vi "Configure Session.vi"(8 "error in":errorcluster, 11 "Plugin in":refnum<class "Statistic.lvclass">) -> (0 "error out":errorcluster, 3 "Plugin out":refnum<class "Statistic.lvclass">)   [LabVIEW 2025, in "Statistic.lvlib" / "Statistic.lvclass"]
uses:
  Statistic.lvclass
  C:/Program Files/National Instruments/LabVIEW 2025/vi.lib/FlexLogger/SDK/PluginSDK.lvlibp/PEFClasses/SDK/Plugin/Plugin.lvclass
  Statistic.lvclass/Statistic.ctl
  <vilib>/FlexLogger/SDK/PluginSDK.lvlibp/PEFClasses/SDK/Producer Channel/Producer Channel.lvclass
  C:/Program Files/National Instruments/LabVIEW 2025/vi.lib/FlexLogger/SDK/PluginSDK.lvlibp/PEFClasses/SDK/Channel/Channel.lvclass
  <vilib>/FlexLogger/SDK/PluginSDK.lvlibp/PEFClasses/SDK/Plugin/ParameterAccess/Read Boolean.vi
  <vilib>/FlexLogger/SDK/PluginSDK.lvlibp/PEFClasses/SDK/Plugin/ParameterAccess/Read DBL.vi
  <vilib>/FlexLogger/SDK/PluginSDK.lvlibp/PEFClasses/SDK/Plugin/ParameterAccess/Read N Channel.vi
  <vilib>/FlexLogger/SDK/PluginSDK.lvlibp/PEFClasses/SDK/Producer Channel/Create Producer Channel_v2.vi
  <vilib>/regexp/Match Regular Expression.xnode
  C:/Program Files/National Instruments/LabVIEW 2025/vi.lib/FlexLogger/SDK/PluginSDK.lvlibp/PEFClasses/SDK/Processing Element/Processing Element.lvclass
  C:/Users/Tester/Documents/LabVIEW Projects/FlexLogger IO Plug-ins/Final Plugins/Statistic/Source/Statistic/Statistic.lvclass
  <vilib>/FlexLogger/SDK/PluginSDK.lvlibp/PEFClasses/SDK/Plugin/Plugin.lvclass
  <vilib>/FlexLogger/SDK/PluginSDK.lvlibp
  kernel32.dll
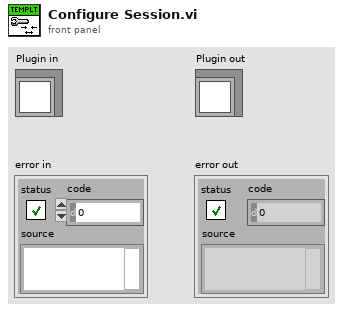
[diagram p1: front panel]
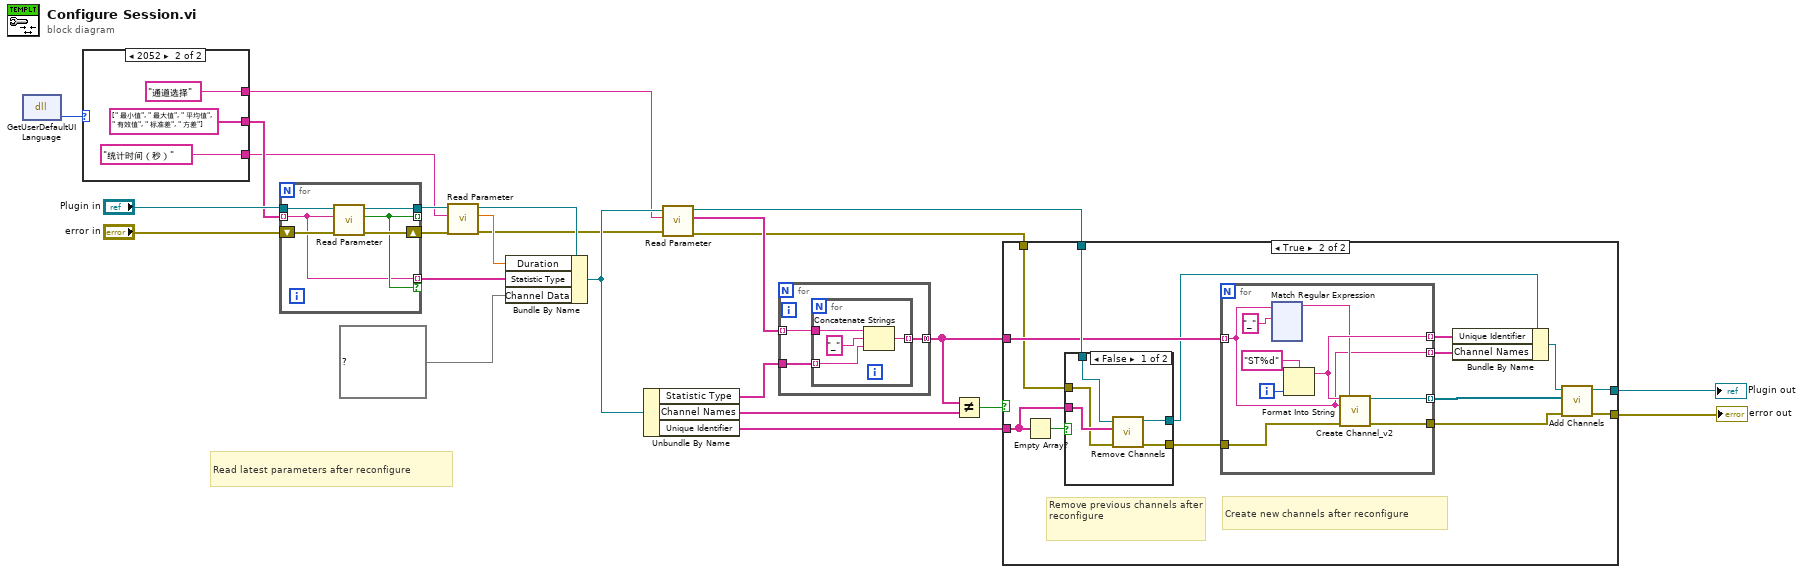
[diagram p0: block diagram]
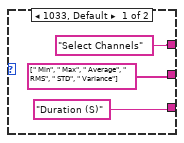
[diagram p2: hidden frame]
diagram:
  # "Read latest parameters after reconfigure"
  n1 = dll-call lib="kernel32.dll" fn="GetUserDefaultUILanguage"() -> ("return type"=w6:u16)  [unwired: 3 in, 2 out]
  n2 = case shown="2052" w6 {
    tunnel: ["Select Channels" ("Name") "通道选择" ("Name")] -> w3
    tunnel: [string[] [" Min", " Max", " Average", " RMS", " STD", " Variance"] ("Unique Identifier") string[] [" 最小值", " 最大值", " 平均值", " 有效值", " 标准差", " 方差"] ("Unique Identifier")] -> w5
    tunnel: ["Duration (S)" ("Name") "统计时间（秒）" ("Name")] -> w4
    frame 1033, Default {
    }
    frame 2052 {
    }
  }
  n3 = for {
    tunnel: "Plugin in" -> [w36]
    tunnel: [w35] -> w17
    tunnel: w5 -> [w31] mode=indexing
    shift-right: [w33] -> w18
    shift-left: "error in" -> [w34]
    tunnel: [w32] -> _ mode=indexing
    tunnel: [w31] -> w20 mode=indexing if=w32
    n4 = call-poly <vilib>:"Read Parameter.vi"("error in (no error)"=w34, "Name"=w31, "Plugin in"=w36) -> ("error out"=w33:errorcluster, "Value"=w32:bool, "Plugin out"=w35:refnum<class "Statistic.lvclass">)  [unwired: 5 in, 1 out]
  }
  n5 = call-poly <vilib>:"Read Parameter.vi"("error in (no error)"=w18, "Name"=w4, "Plugin in"=w17) -> ("error out"=w12:errorcluster, "Value"=w16:dbl, "Plugin out"=w15:refnum<class "Statistic.lvclass">)  [unwired: 5 in, 1 out]
  n6 = Bundle By Name(cluster=w15, "Duration"=w16, "Statistic Type"=w20, "Channel Data"=map{string, dbl[]} {}) -> (w13:refnum<class "Statistic.lvclass">)
  n7 = Unbundle By Name(w13) -> ("Statistic Type"=w19:string[], "Channel Names"=w24:string[], "Unique Identifier"=w22:string[])
  n8 = call-poly <vilib>:"Read Parameter.vi"("error in (no error)"=w12, "Name (Unique Channel Identifier)"=w3, "Plugin in"=w13) -> ("error out"=w9:errorcluster, "Channels"=w11:string[], "Plugin out"=w10:refnum<class "Statistic.lvclass">)  [unwired: 5 in, 1 out]
  n9 = for {
    tunnel: w19 -> [w39]
    tunnel: [w38] -> w21 mode=concatenating
    tunnel: w11 -> [w37] mode=indexing
    n10 = for {
      tunnel: w39 -> [w42] mode=indexing
      tunnel: [w41] -> w38 mode=indexing
      tunnel: w37 -> [w40]
      n11 = Concatenate Strings(w40, "_" ("string"), w42) -> (w41:string)
    }
  }
  n12 = Not Equal?(x=w21, y=w24) -> (x != y?=w23:bool)
  n13 = case shown="True" w23 {
    tunnel: w22 -> [_ w55]
    tunnel: w10 -> [w45 w59]
    tunnel: [w45 w54] -> w2
    tunnel: [w44 w51] -> w1
    tunnel: w21 -> [_ w50]
    tunnel: w9 -> [w44 w46]
    frame False {
    }
    frame True {
      # "Create new channels after reconfigure"
      # "Remove previous channels after reconfigure"
      n14 = Empty Array?(array=w55) -> (empty?=w56:bool)
      n15 = case shown="False" w56 {
        tunnel: w59 -> [w187 w192]
        tunnel: [w190 w191] -> w58
        tunnel: [w189 w192] -> w48
        tunnel: w55 -> [w188 _]
        tunnel: w46 -> [w186 w191]
        frame False {
          n16 = call-dynamic "Remove Channels.vi"("error in (no error)"=w186, "Unique Channel Identifiers to Delete"=w188, "Plugin in"=w187) -> ("error out"=w190:errorcluster, "Plugin out"=w189:refnum<class "Statistic.lvclass">)  [unwired: 7 in]
        }
        frame True {
        }
      }
      n17 = for {
        tunnel: [w67] -> w53 mode=indexing
        tunnel: w58 -> [w68]
        tunnel: [w66] -> w52
        tunnel: [w63] -> w57 mode=indexing
        tunnel: w50 -> [w60] mode=indexing
        tunnel: [w60] -> w49 mode=indexing
        i -> [w64]
        n18 = xnode "Match Regular Expression"("input string"=w60, "regular expression"="_") -> ("before match"=w61:string)  [unwired: 4 in, 4 out]
        n19 = Format Into String(format string="ST%d", w64) -> (resulting string=w63:string)  [unwired: 2 in, 1 out]
        n20 = call-poly <vilib>:"Create Channel_v2.vi"("Unique Channel Identifier"=w63, "Display Group"=w61, "Default Channel Name"=w60, "error in (no error)"=w68) -> ("Producer Channel"=w67:refnum<class "Producer Channel.lvclass">, "error out"=w66:errorcluster)  [unwired: 10 in]
      }
      n21 = Bundle By Name(cluster=w48, "Unique Identifier"=w57, "Channel Names"=w49) -> (w47:refnum<class "Statistic.lvclass">)
      n22 = call <vilib>:"Add Channels.vi"("error in (no error)"=w52, "Channels"=w53, "Plugin in"=w47) -> ("error out"=w51:errorcluster, "Plugin out"=w54:refnum<class "Statistic.lvclass">)  [unwired: 7 in]
    }
  }
  "error out" <- w1
  "Plugin out" <- w2
